vi "Dock Window.vi"(0 "Document in":refnum<class "Document.lvclass">, 5 "Dock?":bool, 7 "Parent Hwnd":i32, 11 "error in (no error)":errorcluster) -> (4 "Document out":refnum<class "Document.lvclass">, 15 "error out":errorcluster)   [LabVIEW 2016, in "Document.lvclass"]
uses:
  Document.lvclass
  Document.lvclass/Document.ctl
  user32.dll
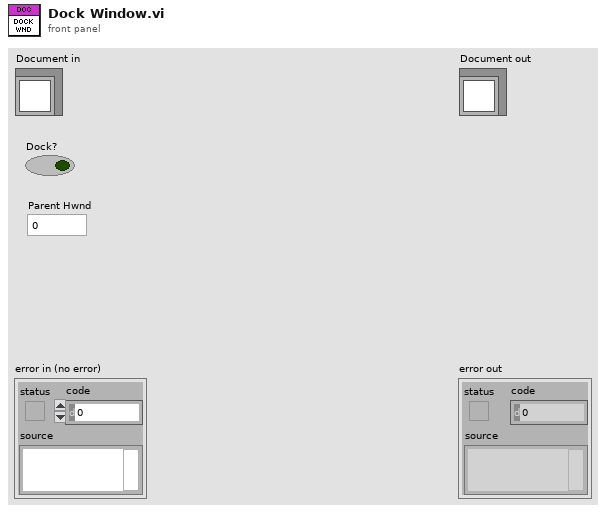
[diagram p1: front panel]
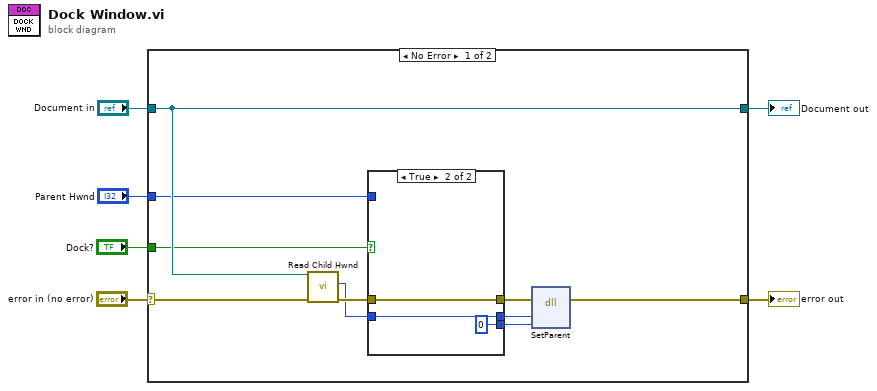
[diagram p0: block diagram]
diagram:
  n1 = case shown="No Error" "error in (no error)" {
    selector: "error in (no error)" -> [w11 w24]
    tunnel: [w10 w24] -> w5
    tunnel: [w9 w23] -> w3
    tunnel: "Document in" -> [w9 w23]
    tunnel: "Dock?" -> [w8 _]
    tunnel: "Parent Hwnd" -> [w7 _]
    frame No Error {
      n2 = call "Read Child Hwnd.vi"("error in (no error)"=w11, "Document in"=w9) -> ("error out"=w13:errorcluster, "Child Hwnd"=w12:u32)  [unwired: 7 in, 1 out]
      n3 = case shown="True" w8 {
        tunnel: w13 -> [w19 w22]
        tunnel: [w19 w22] -> w16
        tunnel: [w18 w21] -> w15
        tunnel: [w17 0 ("hWnd")] -> w14
        tunnel: w12 -> [w18 w21]
        tunnel: w7 -> [w17 _]
        frame False {
        }
        frame True {
        }
      }
      n4 = dll-call lib="user32.dll" fn="SetParent"(error in=w16, "Child"=w15, "NewParent"=w14) -> (error out=w10:errorcluster)  [unwired: 5 in, 1 out]
    }
    frame Error {
    }
  }
  "error out" <- w5
  "Document out" <- w3
